vi "Define Mask.vi"(8 "error in (no error)":errorcluster, 11 "FPGA Image":T3(plugin-control)=refnum) -> (0 "error out":errorcluster)   [LabVIEW 2013]
doc: "GUI for selecting a part type and starting a batch process\nPart types list is passed in from caller.\nReturns when Start or Cancel is pressed."
uses:
  Sectors/Number of Wing Sector.ctl
  Mask ROI FG Enum.ctl
  Mask ROI Cluster.ctl
  Common/File IO/INI/Read write mode.ctl
  Message Passing/MsgQ Loops enum.ctl
  System Status/Status FG Enum.ctl
  Common/State Machines/State Machine Lib.lvlib
  Common/GUI/GUI.lvlib
  <vilib>/vision/NI_Vision_Development_Module.lvlib
  Image Processing.lvlib
  Message Passing/Main MsgQ.lvlib
panel:
  in  "Consecutive \nSector Threshold":u8=5
  in  "Calculate BG":bool
  in  "Load Current Mask":bool
  out "Right ROI":T1={"Global Rectangle"=[696, 31, 1116, 458], "Contours"=[{"ID"=enum."External", "Type"=7, "Coordinates"=[697, 449, 360, 417, 359000, 90000]}]} {"Contours"."Type" items=["No Selection", "Point", "Line", "Rectangle", "Oval", "Polygon", "Freehand Region", "Annulus", "Unused2", "Unused3", "Broken Line", "Freehand Line", "Rotated Rectangle"]}
  out "Left ROI":T1={"Global Rectangle"=[108, 28, 528, 455], "Contours"=[{"ID"=enum."External", "Type"=7, "Coordinates"=[526, 446, 360, 417, 90000, 181000]}]} {"Contours"."Type" items=["No Selection", "Point", "Line", "Rectangle", "Oval", "Polygon", "Freehand Region", "Annulus", "Unused2", "Unused3", "Broken Line", "Freehand Line", "Rotated Rectangle"]}
  out "[Avg BG]":dbl[](array[numeric])=[74.62775735294117, 14.052583862194016, 11.949183303085299, 11.163636363636364, 11.818511796733212, 11.629764065335753, 11.753399818676337, 12.589626933575978, 12.155797101449275, 13.929026387625115, 12.490463215258856, 12.344202898550725, 10.207272727272727, 9.361237488626024, 9.52087114337568, 9.654024051803885, 47.60682226211849, 11.145454545454545, 7.06630336058129, 7.974499089253188, 7.586582048957389, 8.327272727272728, 9.048050770625567, 9.596363636363636, 9.736603088101726, 9.116953762466002, 8.77536231884058, 9.35036496350365, 9.065217391304348, 6.882620564149226, 7.169537624660018, 7.920505871725384]
  in  "NumWingSectors":T2=16 items=["1"=1, "2"=2, "4"=4, "8"=8, "16"=16]
  out "State":string="User Events?"
  in  "Exit":bool
  in  "Save Mask":bool
  out "combo mask":T3(plugin-control)
  out "right mask":T3(plugin-control)
  out "right masked image":T3(plugin-control)
  out "right annulus":T4={"Center X"=697, "Center Y"=449, "Inner Radius"=360, "Outer Radius"=417, "Start Angle"=-1.0, "End Angle"=90.0} {"End Angle" format="%.2f"; "Start Angle" format="%.2f"; "Center X" scale=0.0..1024.0}
  out "left mask":T3(plugin-control)
  out "left masked image":T3(plugin-control)
  out "left annulus":T4={"Center X"=526, "Center Y"=446, "Inner Radius"=360, "Outer Radius"=417, "Start Angle"=90.0, "End Angle"=181.0} {"End Angle" format="%.2f"; "Start Angle" format="%.2f"; "Center X" scale=0.0..1024.0}
  in  "Accept Threshold":bool
  out "Processed Image":T3(plugin-control)
  in  "Threshold Range":cluster{"Lower value":dbl, "Upper value":dbl}={"Lower value"=3.0, "Upper value"=255.0} {"Upper value" min=0.0 max=255.0 scale=0.0..255.0; "Lower value" min=0.0 max=255.0}
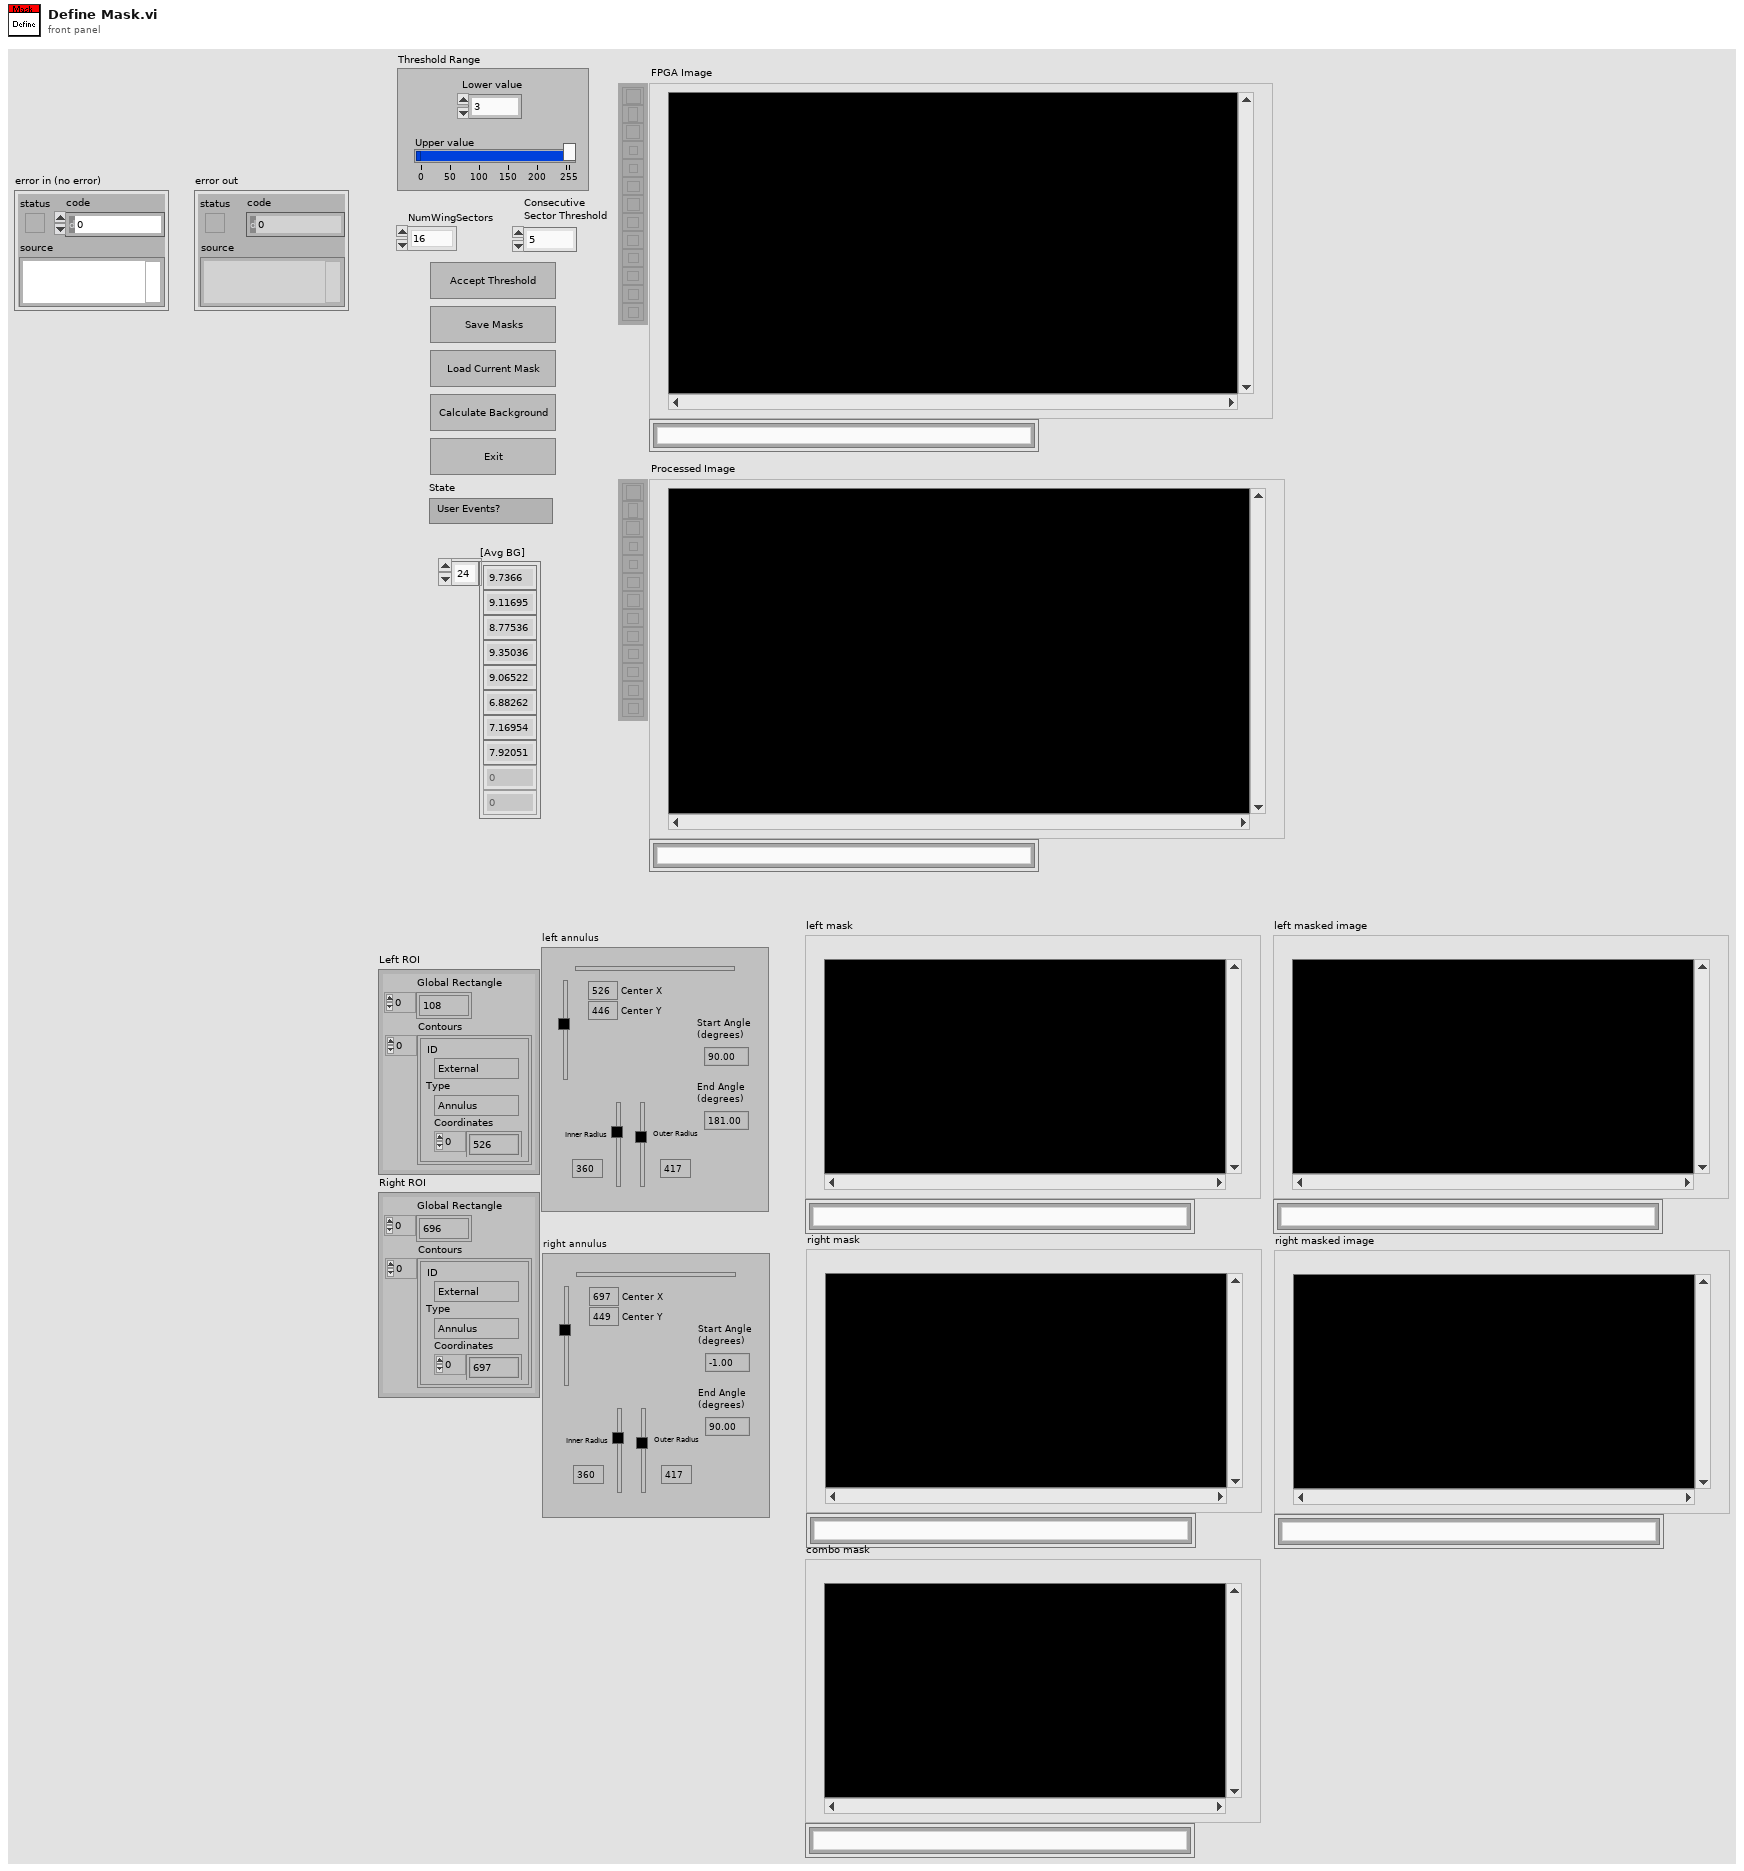
[diagram p1: front panel]
types:
  T1 = typedef "ROI Descriptor" = cluster{"Global Rectangle":i32[], "Contours":cluster{"ID":enum32{"External", "Internal"}, "Type":u32, "Coordinates":i32[]}[]}
  T2 = typedef "Number of Wing Sector.ctl" = u8
  T3 = typedef "IMAQ Image.ctl" = refnum<image>
  T4 = typedef "IMAQ Circle" = cluster{"Center X":i32, "Center Y":i32, "Inner Radius":i32, "Outer Radius":i32, "Start Angle":dbl, "End Angle":dbl}
  T5 = typedef "State Machine Lib.lvlib/STATE cluster.ctl" = cluster{"State":string, "Parameters":variant}
  T6 = typedef "Mask ROI FG Enum.ctl" = enum16{"Read", "Write", "Enable Background", "Disable Background"}
  T7 = typedef "Main MsgQ.lvlib/MsgQ Loops enum.ctl" = enum16{"User Interface", "Image Acq"}
  T8 = typedef "Read write mode.ctl" = enum16{"Read", "Write"}
  T9 = typedef "Mask ROI Cluster.ctl" = cluster{"left annulus":T4, "right annulus":T4, "Threshold Range":cluster{"Lower value":dbl, "Upper value":dbl}, "[Avg BG]":u8[], "Number of Sectors":u8, "Left ROI":T1, "Right ROI":T1, "Left Start Angle Duty Cycle":fxp<+,8,0>, "Left End Angle Duty Cycle":fxp<+,8,0>, "Right End Angle Duty Cycle":fxp<+,8,0>, "Right Start Angle Duty Cycle":fxp<+,8,0>, "[Sector ROIs]":T1[], "Consecutive Sector Threshold":u8}
  T10 = typedef "Status FG Enum.ctl" = enum16{"Reset", "Read", "Write"}
  T11 = typedef "Sector Parameter Cluster.ctl" = cluster{"Start Angle":fxp<+/-,17,2>, "End Angle":fxp<+/-,17,2>, "Inner Radius":u16, "Outter Radius":u16, "Hinge X":u16, "Hinge Y":u16, "NumWingSectors":u8}
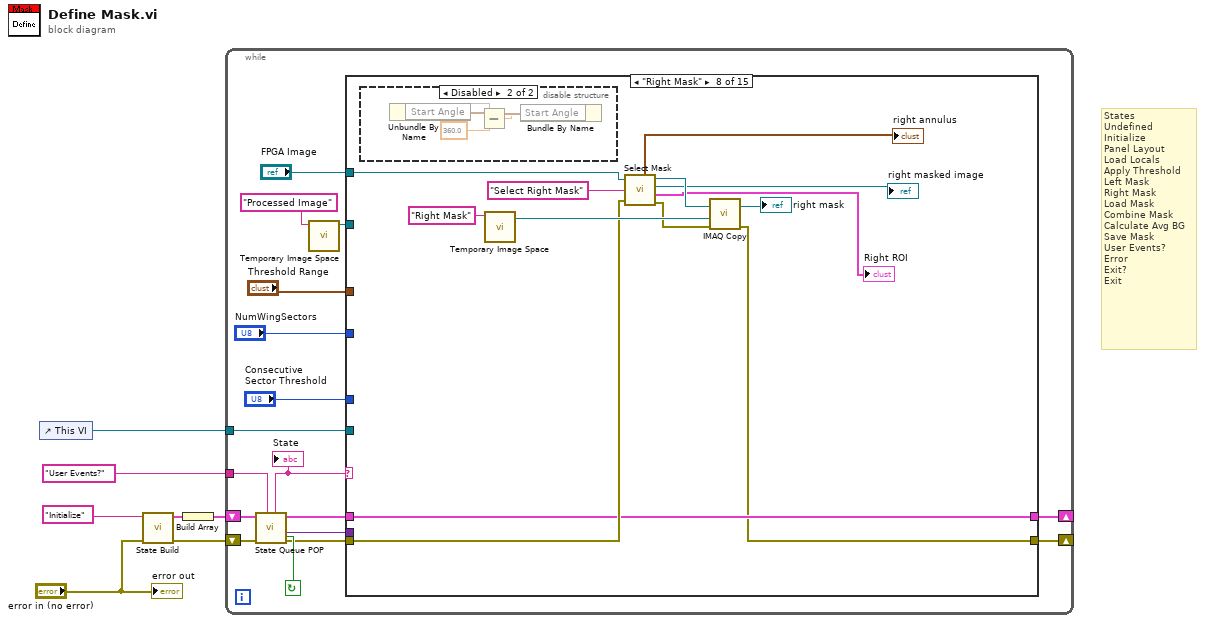
[diagram p0: block diagram]
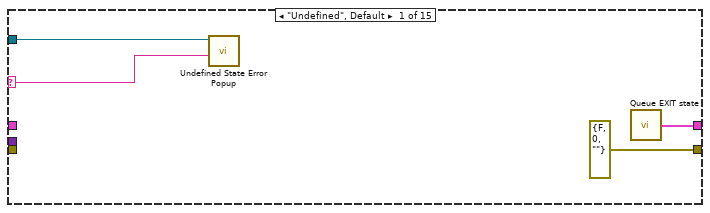
[diagram p2: hidden frame]
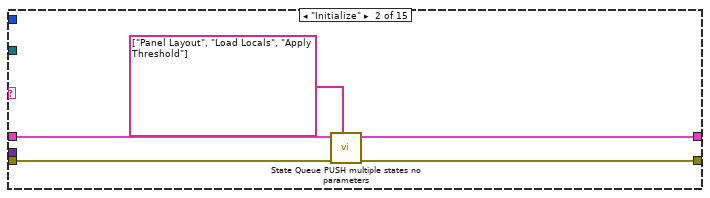
[diagram p3: hidden frame]
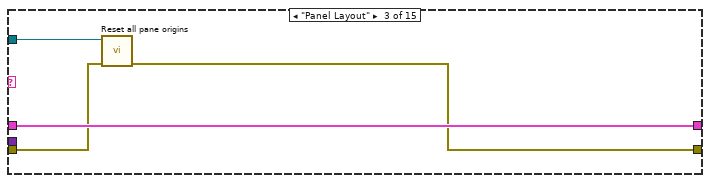
[diagram p4: hidden frame]
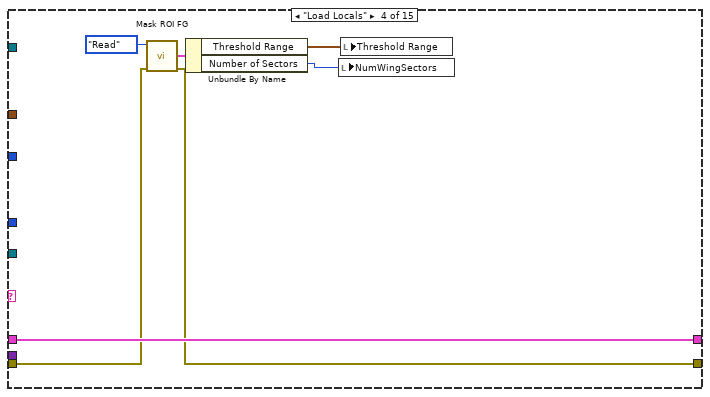
[diagram p5: hidden frame]
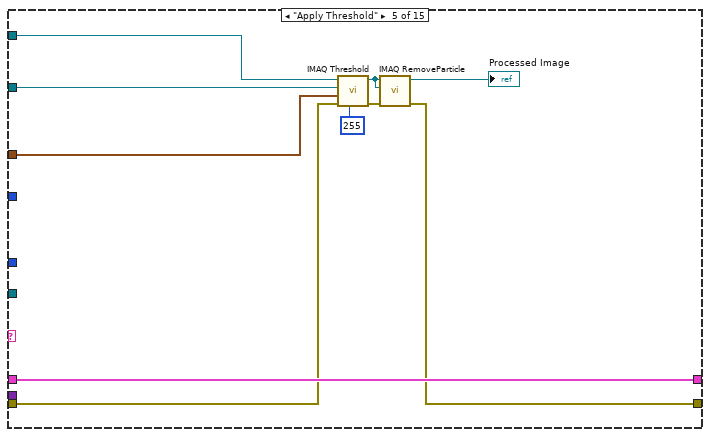
[diagram p6: hidden frame]
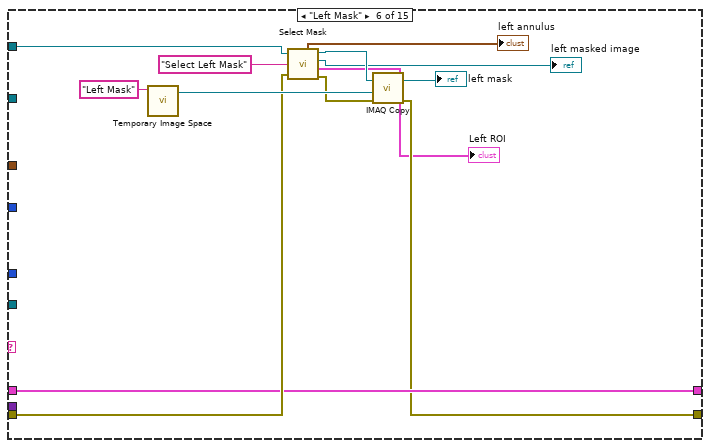
[diagram p7: hidden frame]
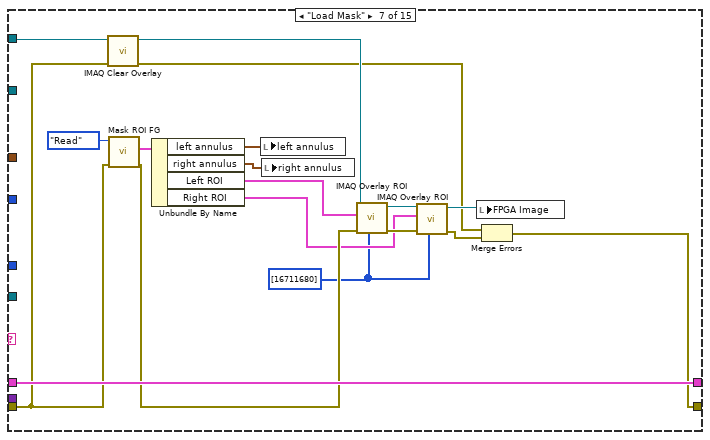
[diagram p8: hidden frame]
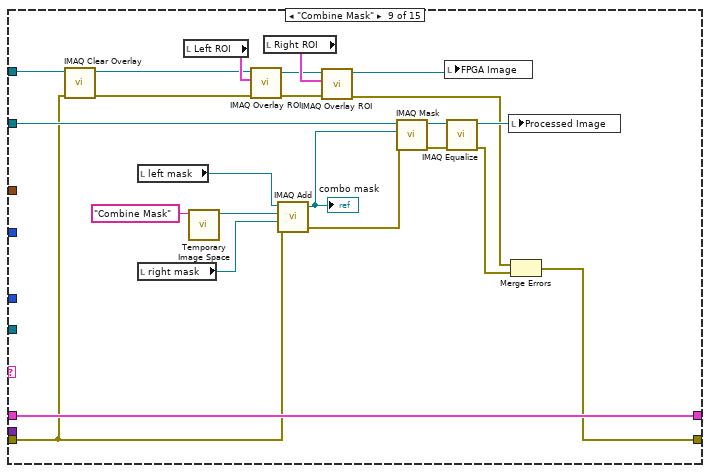
[diagram p10: hidden frame]
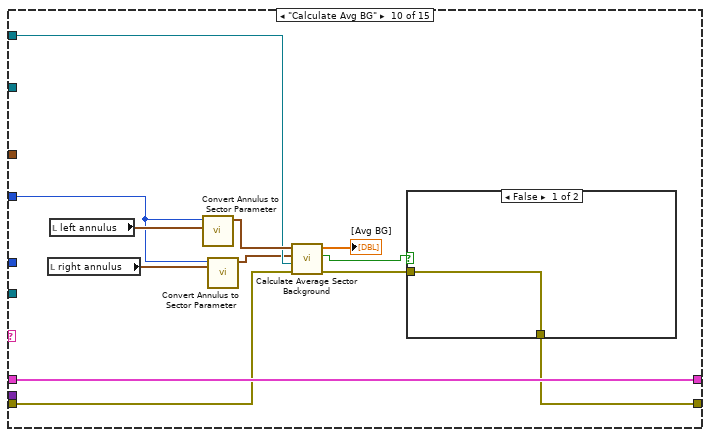
[diagram p11: hidden frame]
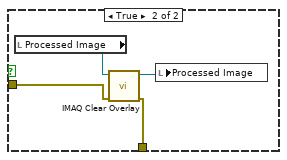
[diagram p12: hidden frame]
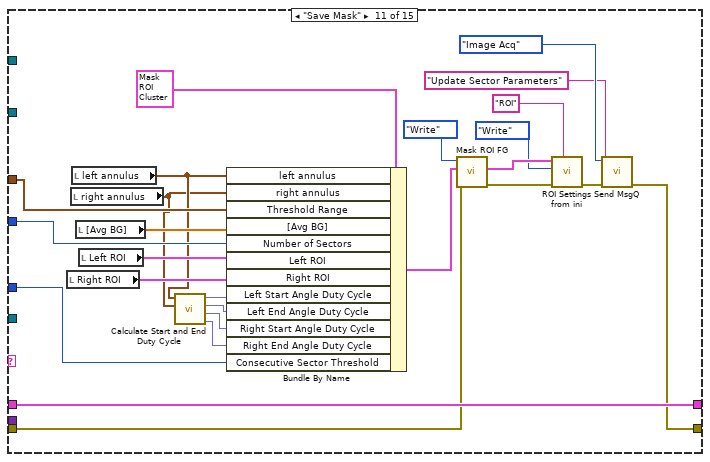
[diagram p13: hidden frame]
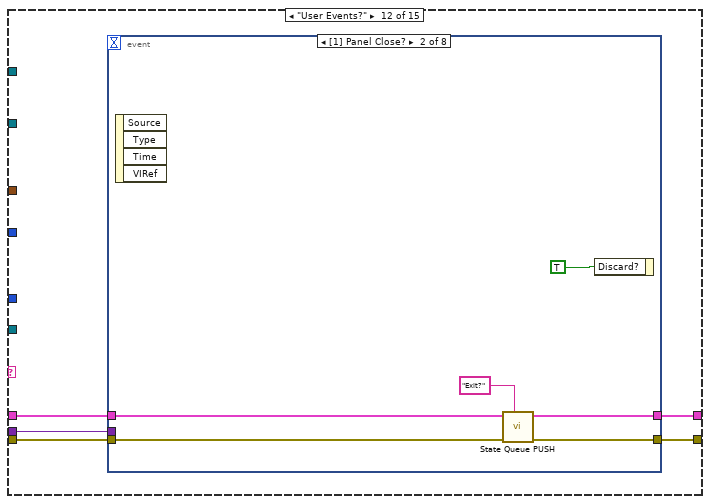
[diagram p14: hidden frame]
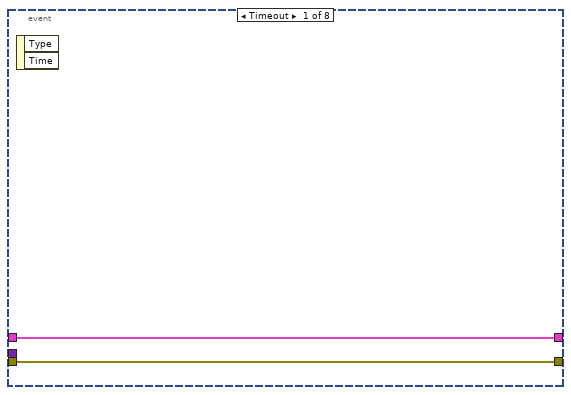
[diagram p15: hidden frame]
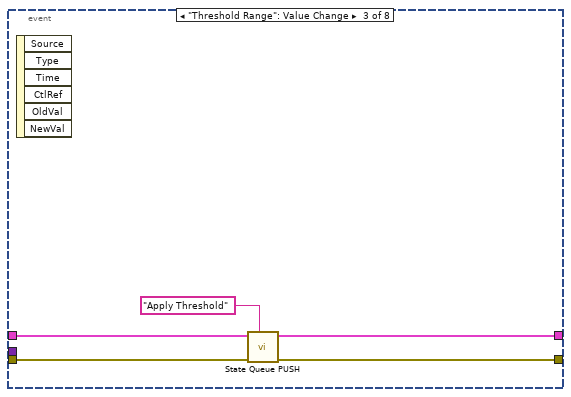
[diagram p16: hidden frame]
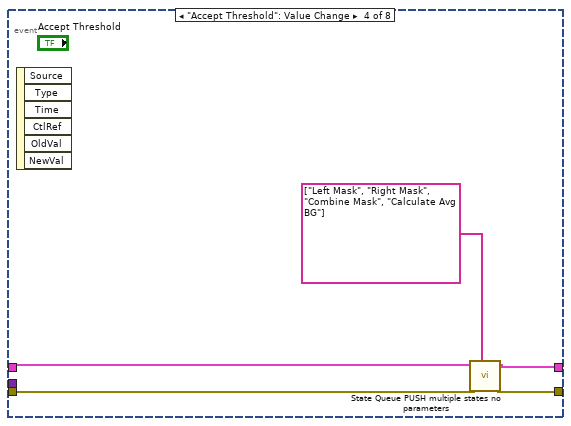
[diagram p17: hidden frame]
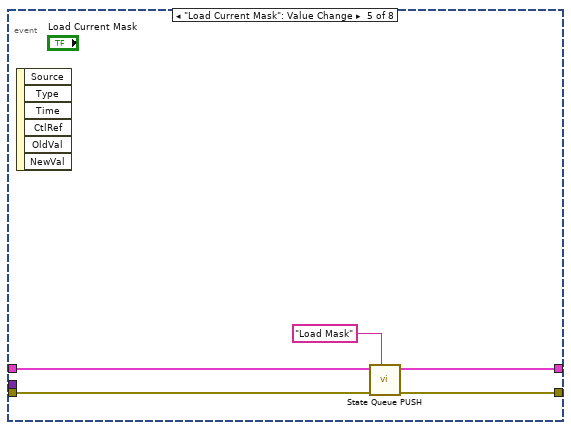
[diagram p18: hidden frame]
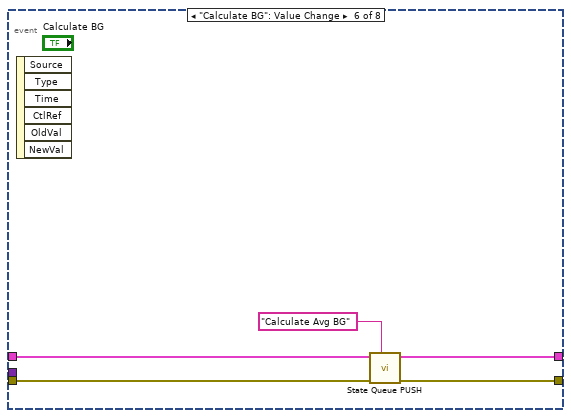
[diagram p19: hidden frame]
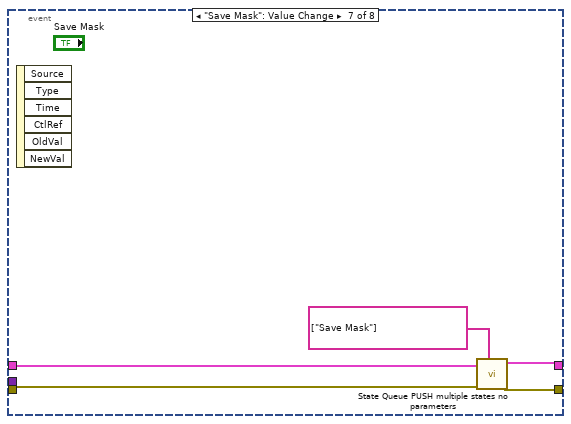
[diagram p20: hidden frame]
diagram:
  # "States\nUndefined\nInitialize\nPanel Layout\nLoad Locals\nApply Threshold\nLeft Mask\nRight Mask\nLoad Mask\nCombine Mask\nCalculate Avg BG\nSave Mask\nUser Events?\nError\nExit?\nExit"
  n1 = control-ref of="This VI"() -> (w6:refnum<vi>)
  n2 = call "State Build.vi"("error in (no error)"="error in (no error)", "State"="Initialize") -> ("error out"=w3:errorcluster, "State Out"=w4:T5)  [unwired: 8 in]
  n3 = Build Array(w4) -> (w5:T5[])
  n4 = while {
    shift-right: [w15] -> _
    shift-left: w3 -> [w23]
    shift-right: [w14] -> _
    shift-left: w5 -> [w21]
    tunnel: "User Events?" ("Default state") -> [w22]
    tunnel: w6 -> [w17]
    stop <- w24 continue-if-true
    n5 = call "State Queue POP.vi"("Default state"=w22, "error in (no error)"=w23, "State que in"=w21) -> ("error out"=w20:errorcluster, "Parameters"=w16:variant, "State que out"=w19:T5[], "Not Exit?"=w24:bool, "State case out"=w18:string)  [unwired: 4 out]
    "State" <- w18
    n6 = call "Temporary Image Space.vi"("Image Name"="Processed Image") -> ("Image Out"=w11:T3)  [unwired: 10 in]
    n7 = case shown="\"Right Mask\"" w18 {
      selector: w18 -> [w25 _ _ _ _ _ _ _ _ _ _ _ _ _ _]
      tunnel: w20 -> [_ w31 w35 w43 w49 w60 w73 w91 w110 w136 w162 w171 w211 w225 w228]
      tunnel: w19 -> [_ w33 w37 w44 w50 w59 w84 w90 w115 w137 w167 w172 _ w219 w230]
      tunnel: w17 -> [w26 _ w36 _ _ _ _ _ _ _ _ _ _ _ _]
      tunnel: w16 -> [_ _ _ _ _ _ _ _ _ _ _ w170 _ _ _]
      tunnel: [errorcluster {"status"=FALSE, "code"=0, "source"=""} ("error out") w32 w34 w38 w48 w58 w68 w89 w103 w127 w152 w169 errorcluster {"status"=FALSE, "code"=0, "source"=""} ("error out") w225 w226] -> w15
      tunnel: [w28 w29 w37 w44 w50 w59 w84 w90 w115 w137 w167 w168 w216 w218 w230] -> w14
      tunnel: "Threshold Range" -> [_ _ _ _ w47 _ _ _ _ _ w164 _ _ _ _]
      tunnel: "FPGA Image" -> [_ _ _ _ w46 w61 w74 w92 w111 w133 _ _ _ _ w229]
      tunnel: w11 -> [_ _ _ _ w45 _ _ _ w118 _ _ _ _ _ _]
      tunnel: "NumWingSectors" -> [_ _ _ _ _ _ _ _ _ w131 w160 _ _ _ _]
      tunnel: "Consecutive \nSector Threshold" -> [_ _ _ _ _ _ _ _ _ _ w143 _ _ _ _]
      frame "Undefined", Default {
        n8 = call "Undefined State Error Popup.vi"("String"=w25, "This VI (Caller if unwired)"=w26) -> ()  [unwired: 10 out]
        n9 = call "Queue EXIT state.vi"() -> ("Exit State Q"=w28:T5[])  [unwired: 1 in]
      }
      frame "Initialize" {
        n10 = call "State Queue PUSH multiple states no parameters.vi"("States to queue"=string[] ["Panel Layout", "Load Locals", "Apply Threshold"], "error in (no error)"=w31, "State que in"=w33) -> ("error out"=w32:errorcluster, "State que out"=w29:T5[])  [unwired: 1 in, 6 out]
      }
      frame "Panel Layout" {
        n11 = call "Reset all pane origins.vi"("error in (no error"=w35, "Vi Ref In"=w36) -> ("error out"=w34:errorcluster)  [unwired: 9 out]
      }
      frame "Load Locals" {
        n12 = call "Mask ROI FG.vi"("error in (no error)"=w43, "Operation"=Mask_ROI_FG_Enum."Read") -> ("error out"=w38:errorcluster, "Mask ROI Out"=w41:T9)  [unwired: 8 in]
        n13 = Unbundle By Name(w41) -> ("Threshold Range"=w40:cluster{"Lower value":dbl, "Upper value":dbl}, "Number of Sectors"=w39:u8)
        n14 = local write "NumWingSectors"(w39) -> ()
        n15 = local write "Threshold Range"(w40) -> ()
      }
      frame "Apply Threshold" {
        n16 = call "IMAQ Threshold"("Replace Value"=u8 255, "error in (no error)"=w49, "Range"=w47, "Image Dst"=w45, "Image Src"=w46) -> ("error out"=w52:errorcluster, "Image Dst Out"=w54:T3)  [unwired: 1 in, 4 out]
        n17 = call "IMAQ RemoveParticle"("error in (no error)"=w52, "Image Dst"=w54, "Image Src"=w54) -> ("error out"=w48:errorcluster, "Image Dst Out"=→"Processed Image":T3)  [unwired: 4 in, 3 out]
      }
      frame "Left Mask" {
        n18 = call "Temporary Image Space.vi"("Image Name"="Left Mask") -> ("Image Out"=w62:T3)  [unwired: 10 in]
        n19 = call "Select Mask.vi"("error in"=w60, "Prompt"="Select Left Mask", "Read \nImage"=w61) -> ("error out"=w57:errorcluster, "ROI Descriptor Out"=→"Left ROI":T1, "Masked \nImage"=→"left masked image":T3, "Annulus"=→"left annulus":T4, "mask"=w65:T3)  [unwired: 1 out]
        n20 = call "IMAQ Copy"("error in (no error)"=w57, "Image Dst"=w62, "Image Src"=w65) -> ("error out"=w58:errorcluster, "Image Dst Out"=→"left mask":T3)  [unwired: 3 in]
      }
      frame "Load Mask" {
        w71 = u32[] [16711680] ("Colors (Green)")
        n21 = call "IMAQ Clear Overlay"("error in (no error)"=w73, "Image"=w74) -> ("error out"=w70:errorcluster, "Image Out"=w72:T3)  [unwired: 8 in]
        n22 = call "Mask ROI FG.vi"("error in (no error)"=w73, "Operation"=Mask_ROI_FG_Enum."Read") -> ("error out"=w77:errorcluster, "Mask ROI Out"=w83:T9)  [unwired: 8 in]
        n23 = Unbundle By Name(w83) -> ("left annulus"=w82:T4, "right annulus"=w81:T4, "Left ROI"=w76:T1, "Right ROI"=w75:T1)
        n24 = local write "left annulus"(w82) -> ()
        n25 = local write "right annulus"(w81) -> ()
        n26 = call "IMAQ Overlay ROI"("Colors (Green)"=w71, "error in (no error)"=w77, "ROI Descriptor"=w76, "Image"=w72) -> ("error out"=w78:errorcluster, "Image Out"=w80:T3)  [unwired: 6 in]
        n27 = call "IMAQ Overlay ROI"("Colors (Green)"=w71, "error in (no error)"=w78, "ROI Descriptor"=w75, "Image"=w80) -> ("error out"=w69:errorcluster, "Image Out"=w79:T3)  [unwired: 6 in]
        n28 = local write "FPGA Image"(w79) -> ()
        n29 = Merge Errors(w70, w69) -> (w68:errorcluster)
      }
      frame "Right Mask" {
        n30 = disable-structure shown="Disabled" {
          frame Enabled {
          }
          frame Disabled {
            n31 = Unbundle By Name() -> (w102:T4, "Start Angle"=w99)
            n32 = Subtract(x=w99, y=360.0) -> (x-y=w101:dbl)
            n33 = Bundle By Name(cluster=w102, "Start Angle"=w101) -> ()  [unwired: 1 out]
          }
        }
        n34 = call "Temporary Image Space.vi"("Image Name"="Right Mask") -> ("Image Out"=w93:T3)  [unwired: 10 in]
        n35 = call "Select Mask.vi"("error in"=w91, "Prompt"="Select Right Mask", "Read \nImage"=w92) -> ("error out"=w88:errorcluster, "ROI Descriptor Out"=→"Right ROI":T1, "Masked \nImage"=→"right masked image":T3, "Annulus"=→"right annulus":T4, "mask"=w96:T3)  [unwired: 1 out]
        n36 = call "IMAQ Copy"("error in (no error)"=w88, "Image Dst"=w93, "Image Src"=w96) -> ("error out"=w89:errorcluster, "Image Dst Out"=→"right mask":T3)  [unwired: 3 in]
      }
      frame "Combine Mask" {
        n37 = call "IMAQ Clear Overlay"("error in (no error)"=w110, "Image"=w111) -> ("error out"=w109:errorcluster, "Image Out"=w108:T3)  [unwired: 8 in]
        n38 = local read "left mask"() -> (w120:T3)
        n39 = local read "right mask"() -> (w119:T3)
        n40 = local read "Left ROI"() -> (w114:T1)
        n41 = call "Temporary Image Space.vi"("Image Name"="Combine Mask") -> ("Image Out"=w122:T3)  [unwired: 10 in]
        n42 = call "IMAQ Overlay ROI"("error in (no error)"=w109, "ROI Descriptor"=w114, "Image"=w108) -> ("error out"=w107:errorcluster, "Image Out"=w106:T3)  [unwired: 7 in]
        n43 = local read "Right ROI"() -> (w113:T1)
        n44 = call "IMAQ Add"("Image Src A"=w120, "Image Dst"=w122, "Image Src B"=w119, "error in (no error)"=w110) -> ("Image Dst Out"=w123:T3, "error out"=w116:errorcluster)  [unwired: 3 in]
        "combo mask" <- w123
        n45 = call "IMAQ Overlay ROI"("error in (no error)"=w107, "ROI Descriptor"=w113, "Image"=w106) -> ("error out"=w105:errorcluster, "Image Out"=w112:T3)  [unwired: 7 in]
        n46 = call "IMAQ Mask"("error in (no error)"=w116, "Image Mask"=w123, "Image Src"=w118) -> ("error out"=w124:errorcluster, "Image Dst Out"=w125:T3)  [unwired: 1 in, 1 out]
        n47 = local write "FPGA Image"(w112) -> ()
        n48 = call "IMAQ Equalize"("error in (no error)"=w124, "Image Src"=w125) -> ("error out"=w104:errorcluster, "Image Dst Out"=w117:T3)  [unwired: 4 in, 4 out]
        n49 = local write "Processed Image"(w117) -> ()
        n50 = Merge Errors(w105, w104) -> (w103:errorcluster)
      }
      frame "Calculate Avg BG" {
        n51 = local read "right annulus"() -> (w130:T4)
        n52 = local read "left annulus"() -> (w135:T4)
        n53 = call "Convert Annulus to Sector Parameter.vi"("Annulus"=w135, "NumWingSectors"=w131) -> ("Sector Parameter"=w134:T11)  [unwired: 9 in]
        n54 = call "Convert Annulus to Sector Parameter.vi"("Annulus"=w130, "NumWingSectors"=w131) -> ("Sector Parameter"=w129:T11)  [unwired: 9 in]
        n55 = call "Calculate Average Sector Background.vi"("error in (no error)"=w136, "Image"=w133, "Right Sector Parameters"=w129, "Left Sector Parameters"=w134) -> ("error out"=w128:errorcluster, "Canceled?"=w126:bool, "[Avg BG]"=→"[Avg BG]":dbl[])  [unwired: 5 in]
        n56 = case shown="False" w126 {
          tunnel: w128 -> [w138 w141]
          tunnel: [w138 w140] -> w127
          frame False {
          }
          frame True {
            n57 = local read "Processed Image"() -> (w142:T3)
            n58 = call "IMAQ Clear Overlay"("error in (no error)"=w141, "Image"=w142) -> ("error out"=w140:errorcluster, "Image Out"=w139:T3)  [unwired: 8 in]
            n59 = local write "Processed Image"(w139) -> ()
          }
        }
      }
      frame "Save Mask" {
        n60 = local read "Right ROI"() -> (w150:T1)
        n61 = local read "right annulus"() -> (w148:T4)
        n62 = local read "left annulus"() -> (w149:T4)
        n63 = local read "[Avg BG]"() -> (w161:dbl[])
        n64 = local read "Left ROI"() -> (w151:T1)
        n65 = call "Calculate Start and End Duty Cycle.vi"("right annulus"=w148, "left annulus"=w149) -> ("Right End Angle Duty Cycle"=w144:fxp<+,8,0>, "Right Start Angle Duty Cycle"=w145:fxp<+,8,0>, "Left End Angle Duty Cycle"=w146:fxp<+,8,0>, "Left Start Angle Duty Cycle"=w147:fxp<+,8,0>)  [unwired: 6 in]
        n66 = Bundle By Name(cluster=T9 {"left annulus"={"Center X"=929, "Center Y"=663, "Inner Radius"=200, "Outer Radius"=405, "Start Angle"=90.0, "End Angle"=180.0}, "right annulus"={"Center X"=929, "Center Y"=663, "Inner Radius"=200, "Outer Radius"=405, "Start Angle"=90.0, "End Angle"=180.0}, "Threshold Range"={"Lower value"=106.82432432432432, "Upper value"=255.0}, "[Avg BG]"=[], "Number of Sectors"=0, "Left ROI"={"Global Rectangle"=[], "Contours"=[]}, "Right ROI"={"Global Rectangle"=[], "Contours"=[]}, "Left Start Angle Duty Cycle"=0.0, "Left End Angle Duty Cycle"=0.0, "Right End Angle Duty Cycle"=0.0, "Right Start Angle Duty Cycle"=0.0, "[Sector ROIs]"=[], "Consecutive Sector Threshold"=0} ("Mask ROI In"), "left annulus"=w149, "right annulus"=w148, "Threshold Range"=w164, "[Avg BG]"=w161, "Number of Sectors"=w160, "Left ROI"=w151, "Right ROI"=w150, "Left Start Angle Duty Cycle"=w147, "Left End Angle Duty Cycle"=w146, "Right Start Angle Duty Cycle"=w145, "Right End Angle Duty Cycle"=w144, "Consecutive Sector Threshold"=w143) -> (w163:T9)
        n67 = call "Mask ROI FG.vi"("error in (no error)"=w162, "Mask ROI In"=w163, "Operation"=Mask_ROI_FG_Enum."Write") -> ("error out"=w157:errorcluster, "Mask ROI Out"=w159:T9)  [unwired: 7 in]
        n68 = call "ROI Settings from ini.vi"("Section"="ROI", "error in (no error)"=w157, "Operation"=Read_write_mode."Write", "Mask ROI In"=w159) -> ("error out"=w153:errorcluster)  [unwired: 5 in, 2 out]
        n69 = call "Send MsgQ.vi"("error in (no error)"=w153, "Message String"="Update Sector Parameters", "Send to MsgQ"=MsgQ_Loops_enum."Image Acq") -> ("error out"=w152:errorcluster)  [unwired: 8 in]
      }
      frame "User Events?" {
        n70 = event shown="[1] Panel Close?" {
          selector: _ -> [_ _ _ _ _ _ _ _]
          dyn-events: _ -> [_ _ _ _ _ _ _ _]
          timeout: _ -> [_ _ _ _ _ _ _ _]
          tunnel: w172 -> [w173 w179 w185 w188 w194 w199 w204 w207]
          tunnel: w171 -> [w174 w178 w184 w186 w191 w196 w201 w208]
          tunnel: w170 -> [_ _ _ _ _ _ _ _]
          tunnel: [w174 w176 w182 w189 w192 w197 w202 w209] -> w169
          tunnel: [w173 w177 w183 w190 w193 w198 w203 w210] -> w168
          event Timeout {
            n71 = event-data() -> ()  [unwired: 3 out]
          }
          event Panel Close? {
            n72 = event-data() -> ()  [unwired: 5 out]
            n73 = call "State Queue PUSH.vi"("State case"="Exit?", "error in (no error)"=w178, "State que in"=w179) -> ("error out"=w176:errorcluster, "State que out"=w177:T5[])  [unwired: 2 in, 5 out]
            n74 = event-data("Discard?"=TRUE) -> ()  [unwired: 1 in, 1 out]
          }
          event "Threshold Range": Value Change {
            n75 = event-data() -> ()  [unwired: 7 out]
            n76 = call "State Queue PUSH.vi"("State case"="Apply Threshold", "error in (no error)"=w184, "State que in"=w185) -> ("error out"=w182:errorcluster, "State que out"=w183:T5[])  [unwired: 2 in, 5 out]
          }
          event "Accept Threshold": Value Change {
            n77 = event-data() -> ()  [unwired: 7 out]
            n78 = call "State Queue PUSH multiple states no parameters.vi"("States to queue"=string[] ["Left Mask", "Right Mask", "Combine Mask", "Calculate Avg BG"], "error in (no error)"=w186, "State que in"=w188) -> ("error out"=w189:errorcluster, "State que out"=w190:T5[])  [unwired: 7 in]
          }
          event "Load Current Mask": Value Change {
            n79 = event-data() -> ()  [unwired: 7 out]
            n80 = call "State Queue PUSH.vi"("State case"="Load Mask", "error in (no error)"=w191, "State que in"=w194) -> ("error out"=w192:errorcluster, "State que out"=w193:T5[])  [unwired: 2 in, 5 out]
          }
          event "Calculate BG": Value Change {
            n81 = event-data() -> ()  [unwired: 7 out]
            n82 = call "State Queue PUSH.vi"("State case"="Calculate Avg BG", "error in (no error)"=w196, "State que in"=w199) -> ("error out"=w197:errorcluster, "State que out"=w198:T5[])  [unwired: 2 in, 5 out]
          }
          event "Save Mask": Value Change {
            n83 = event-data() -> ()  [unwired: 7 out]
            n84 = call "State Queue PUSH multiple states no parameters.vi"("States to queue"=string[] ["Save Mask"], "error in (no error)"=w201, "State que in"=w204) -> ("error out"=w202:errorcluster, "State que out"=w203:T5[])  [unwired: 7 in]
          }
          event "Exit": Value Change {
            n85 = event-data() -> ()  [unwired: 7 out]
            n86 = call "State Queue PUSH.vi"("State case"="Exit?", "error in (no error)"=w208, "State que in"=w207) -> ("error out"=w209:errorcluster, "State que out"=w210:T5[])  [unwired: 7 in]
          }
        }
      }
      frame "Error" {
        # "DEFAULT IS \nTO CLEAR ERROR\nAND EXIT"
        n87 = Unbundle By Name(w211) -> ("source"=w214:string)
        n88 = Concatenate Strings("Error: " ("string"), w214) -> (w213:string)
        n89 = call "Status FG.vi"("Status In"=w213, "Operation"=Status_FG_Enum."Write") -> ()  [unwired: 8 in, 2 out]
        n90 = call <vilib>:"Clear Errors.vi"("error in (no error)"=w211) -> ()  [unwired: 7 out]
        n91 = call "Queue EXIT state.vi"() -> ("Exit State Q"=w216:T5[])  [unwired: 1 in]
      }
      frame "Exit?" {
        n92 = Two Button Dialog(message="Exit?", 1:"No" ("F button name (\"Cancel\")"), 2:"Yes" ("T button name (\"OK\")")) -> (T button?=w221:bool)
        n93 = call "Queue EXIT state.vi"() -> ("Exit State Q"=w220:T5[])  [unwired: 1 in]
        n94 = Select(t=w220, s=w221, f=w219) -> (s? t:f=w218:T5[])
      }
      frame "Exit" {
        n95 = call "IMAQ Clear Overlay"("error in (no error)"=w228, "Image"=w229) -> ("error out"=w227:errorcluster)  [unwired: 8 in, 1 out]
        n96 = call <vilib>:"Clear Errors.vi"("error in (no error)"=w227) -> ("error out"=w226:errorcluster)  [unwired: 6 in]
      }
    }
  }
  "error out" <- "error in (no error)"
